vi "Send to Open Instruments.vi"(8 "error in (no error)":errorcluster, 9 "Command":string=": Exit", 10 "Instrument Names":string[](array[string]), 11 "Master":refnum<queue>) -> (0 "error out":errorcluster)   [LabVIEW 2013]
uses:
  MeasurementControl Message Queue Folder/Message Cluster.ctl
  MeasurementControl Message Queue Folder/MeasurementControl Message Queue.lvlib
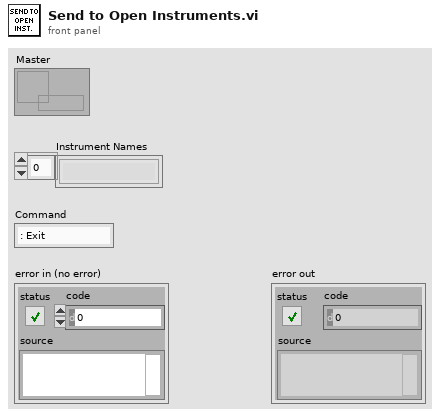
[diagram p1: front panel]
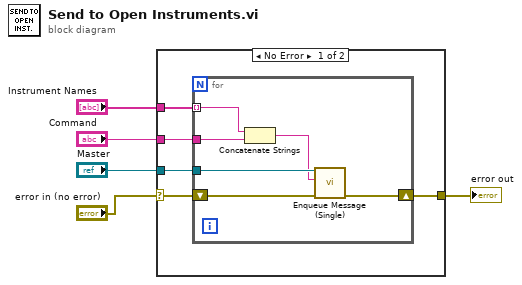
[diagram p0: block diagram]
diagram:
  n1 = case shown="No Error" "error in (no error)" {
    selector: "error in (no error)" -> [w7 w17]
    tunnel: "Instrument Names" -> [w10 _]
    tunnel: "Master" -> [w9 _]
    tunnel: [w8 w17] -> w2
    tunnel: "Command" -> [w6 _]
    frame No Error {
      n2 = for {
        tunnel: w10 -> [w16] mode=indexing
        tunnel: w9 -> [w15]
        shift-right: [w13] -> w8
        shift-left: w7 -> [w12]
        tunnel: w6 -> [w11]
        n3 = Concatenate Strings(w16, w11) -> (w14:string)
        n4 = call "Enqueue Message (Single).vi"("error in (no error)"=w12, "Message"=w14, "Message Queue"=w15) -> ("error out"=w13:errorcluster)  [unwired: 7 in, 1 out]
      }
    }
    frame Error {
    }
  }
  "error out" <- w2
